vi "Check Multiple Uses same HW Configuration File.vi"(8 "error in (no error)":errorcluster, 11 "Item Ref in":T1 format="%.0x") -> (0 "error out":errorcluster)   [LabVIEW 2020, in "Ballard 1553 System Explorer.lvlib"]
uses:
  Ballard 1553 System Explorer.lvlib
  <vilib>/NI VeriStand/Custom Device API/Custom Device Item Ref.ctl
  Shared/Controls and Global/Global.vi
  <vilib>/NI VeriStand/Custom Device Tools/Custom Device Utility Library/NI VeriStand - Search for All Items by GUID.vi
  <vilib>/NI VeriStand/Custom Device API/Get Item Property (Path).vi
  <userlib>/_OpenG.lib/md5/md5.llb/MD5 Message Digest (Binary String)__ogtk.vi
  <userlib>/_OpenG.lib/array/array.llb/Remove Duplicates from 1D Array (String)__ogtk.vi
  <vilib>/NI VeriStand/Custom Device API/Custom Device API.lvlib
  <vilib>/NI VeriStand/Custom Device Tools/Custom Device Utility Library/Custom Device Utility Library.lvlib
  Shared/Ballard 1553 Shared.lvlib
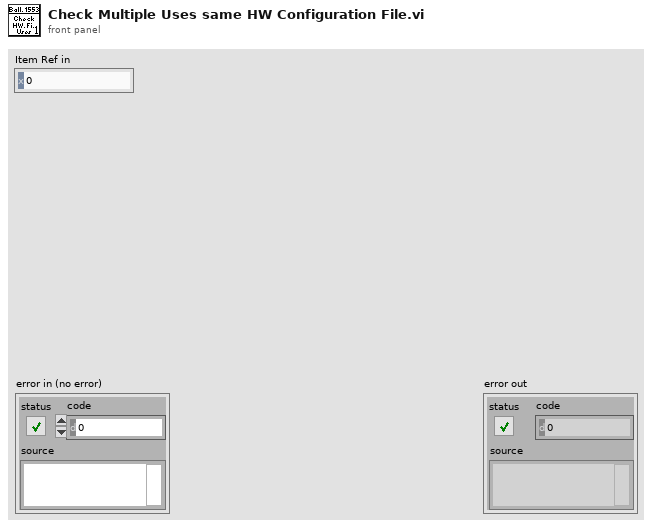
[diagram p1: front panel]
types:
  T1 = typedef "Custom Device API.lvlib/Custom Device Item Ref.ctl" = u64
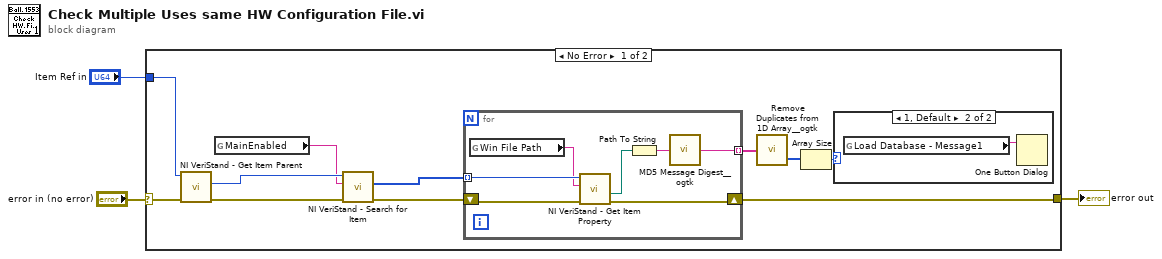
[diagram p0: block diagram]
diagram:
  n1 = case shown="No Error" "error in (no error)" {
    selector: "error in (no error)" -> [w14 w23]
    tunnel: [w6 w23] -> w2
    tunnel: "Item Ref in" -> [w13 _]
    frame No Error {
      n2 = call <vilib>:"NI VeriStand - Get Item Parent.vi"("error in (no error)"=w14, "Item Ref in"=w13) -> ("error out"=w12:errorcluster, "Parent Ref"=w11:T1)  [unwired: 6 in, 2 out]
      n3 = global read "Global.vi" "MainEnabled"() -> (w4:string)
      n4 = call-poly <vilib>:"NI VeriStand - Search for Item.vi"("error in"=w12, "Item GUID"=w4, "Section Ref in"=w11) -> ("error out"=w9:errorcluster, "Item Refs"=w10:T1[])  [unwired: 5 in, 2 out]
      n5 = for {
        tunnel: w10 -> [w22] mode=indexing
        shift-right: [w19] -> w6
        shift-left: w9 -> [w21]
        tunnel: [w17] -> w8 mode=indexing
        n6 = global read "Global.vi" "Win File Path"() -> (w16:string)
        n7 = call-poly <vilib>:"NI VeriStand - Get Item Property.vi"("error in (no error)"=w21, "Property Name"=w16, "Item Ref in"=w22) -> ("error out"=w19:errorcluster, "Value"=w20:path)  [unwired: 5 in, 2 out]
        n8 = Path To String(path=w20) -> (string=w18:string)
        n9 = call-poly <userlib>:"MD5 Message Digest__ogtk.vi"("Message"=w18) -> ("MD5 Message Digest"=w17:string)
      }
      n10 = call-poly <userlib>:"Remove Duplicates from 1D Array__ogtk.vi"("Input Array"=w8) -> ("indices of removed elements"=w7:i32[])  [unwired: 1 out]
      n11 = Array Size(array=w7) -> (size(s)=w5:i32)
      n12 = case shown="1, Default" w5 {
        frame 0 {
        }
        frame 1, Default {
          n13 = global read "Global.vi" "Load Database - Message1"() -> (w15:string)
          n14 = One Button Dialog(message=w15) -> ()  [unwired: 1 in, 1 out]
        }
      }
    }
    frame Error {
    }
  }
  "error out" <- w2
